vi "xijk_average_non_zeros.vi"(9 "threshold":sgl, 11 "array in":sgl[](array[numeric])) -> (3 "average over non-zeros":sgl)   [LabVIEW 2009]
uses:
  <vilib>/Analysis/8numeric.llb/1D Numeric Integration.vi
  <vilib>/Analysis/NI_AALPro.lvlib
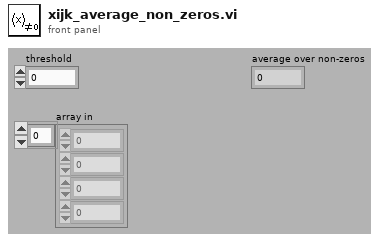
[diagram p1: front panel]
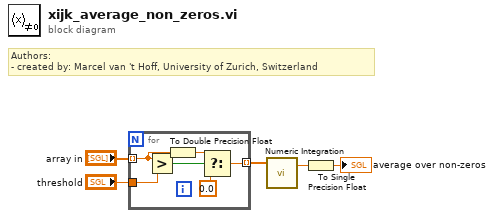
[diagram p0: block diagram]
diagram:
  # "Authors: \n- created by: Marcel van 't Hoff, University of Zurich, Switzerland"
  n1 = for {
    tunnel: "array in" -> [w10] mode=indexing
    tunnel: "threshold" -> [w11]
    tunnel: [w7] -> w2 mode=indexing
    n2 = Greater?(x=w10, y=w11) -> (0:w9:bool)
    n3 = To Double Precision Float(number=w10) -> (double precision float=w6:dbl)
    n4 = Select(t=w6, s=w9, f=0.0 ("t")) -> (s? t:f=w7:dbl)
  }
  n5 = call-poly <vilib>:"Numeric Integration.vi"("Input Array"=w2) -> ("result"=w1:dbl)  [unwired: 2 in, 1 out]
  n6 = To Single Precision Float(number=w1) -> (single precision float=→"average over non-zeros":sgl)
